vi "NIVS Reference Write .vi"(4 "error in (no error)":errorcluster, 5 "Value":refnum<k24>, 6 "Container State":T4, 7 "Display State In":T1={"Initialization"=TRUE, "Show In and out values"=TRUE, "Show Highliting"=TRUE, "Open Plot"=FALSE, "Format String"="%10_4g", "X"=0.0, "Limits"={"Min X"=-inf, "Max X"=inf, "MaxDiff X"=inf, "MaxGrad X"=inf, "Min Y"=-inf, "Max Y"=inf, "MaxDiff Y"=inf}, "Vertical Scrollbar"=FALSE, "Data"={"X"=[0.0, 5.0], "Y"=[0.0, 100.0]}, "Undo Avaliable"=FALSE, "NIVS.System Definition Root"=refnum}) -> (0 "error out":errorcluster, 3 "Display State Out":T1={"Initialization"=TRUE, "Show In and out values"=TRUE, "Show Highliting"=TRUE, "Open Plot"=FALSE, "Format String"="%10_4g", "X"=0.0, "Limits"={"Min X"=-inf, "Max X"=inf, "MaxDiff X"=inf, "MaxGrad X"=inf, "Min Y"=-inf, "Max Y"=inf, "MaxDiff Y"=inf}, "Vertical Scrollbar"=FALSE, "Data"={"X"=[0.0, 5.0], "Y"=[0.0, 100.0]}, "Undo Avaliable"=FALSE, "NIVS.System Definition Root"=refnum})   [LabVIEW 2011]
uses:
  <vilib>/_xctls/Container State.ctl
  State TBL1D.ctl
  Limits TBL1D.ctl
  Data TBL1D.ctl
  NationalInstruments.VeriStand.SystemStorage
  <vilib>/_xctls/XControlSupport.lvlib
  TBL1D.xctl
panel:
  in  "Value":bool
  # "Replace the Value Control below with a Control of desired type.\nDo not remove this Control or the others from the connector pane.\nDo not change the connector pane pattern.\nThe Value control should always be the third terminal from top on the input side in the connector pane."
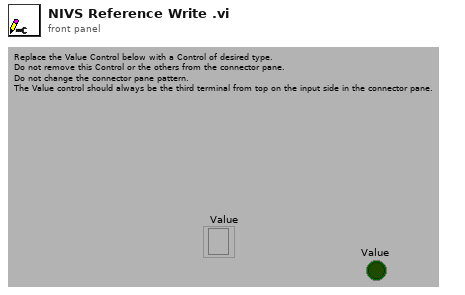
[diagram p1: front panel]
types:
  T1 = typedef "TBL1D.xctl/State TBL1D.ctl" = cluster{"Initialization":bool, "Show In and out values":bool, "Show Highliting":bool, "Open Plot":bool, "Format String":string, "X":sgl, "Limits":T2, "Vertical Scrollbar":bool, "Data":T3, "Undo Avaliable":bool, "NIVS.System Definition Root":refnum<k24>}
  T2 = typedef "TBL1D.xctl/Limits TBL1D.ctl" = cluster{"Min X":sgl, "Max X":sgl, "MaxDiff X":sgl, "MaxGrad X":sgl, "Min Y":sgl, "Max Y":sgl, "MaxDiff Y":sgl}
  T3 = typedef "TBL1D.xctl/Data TBL1D.ctl" = cluster{"X":sgl[], "Y":sgl[]}
  T4 = typedef "XControlSupport.lvlib/Container State.ctl" = cluster{"Indicator?":bool, "Run Mode?":bool, " Refnum":refnum<vi>}
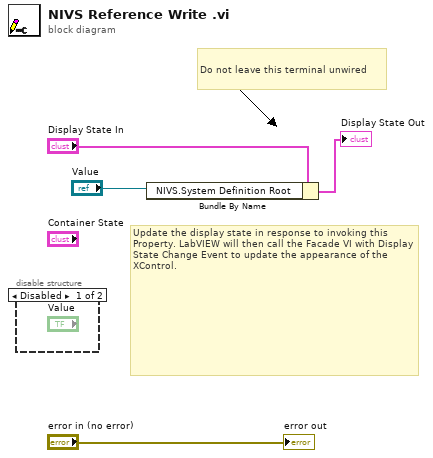
[diagram p0: block diagram]
diagram:
  # "Do not leave this terminal unwired"
  # "Update the display state in response to invoking this Property. LabVIEW will then call the Facade VI with Display State Change Event to update the appearance of the XControl."
  n1 = disable-structure shown="Disabled" {
    frame Disabled {
    }
    frame Enabled {
    }
  }
  n2 = Bundle By Name(cluster="Display State In", "NIVS.System Definition Root"="Value") -> (→"Display State Out":T1)
  "error out" <- "error in (no error)"
